vi "Set Workbook.vi"(8 "error in (no error)":errorcluster, 10 "Workbook":refnum<k24>, 11 "Excel Legacy in":refnum<class "Excel Legacy.lvclass">) -> (0 "error out":errorcluster, 3 "Excel Legacy out":refnum<class "Excel Legacy.lvclass">)   [LabVIEW 2013, in "Excel Legacy.lvclass"]
uses:
  Excel Legacy.lvclass
  Excel Legacy.lvclass/Excel Legacy.ctl
  C:/PhaeronGit/LVNPOI/Resources/NPOI 2.1.1 dotnet2/NPOI.dll
  Resources/NPOI 2.1.1 dotnet2/NPOI.dll
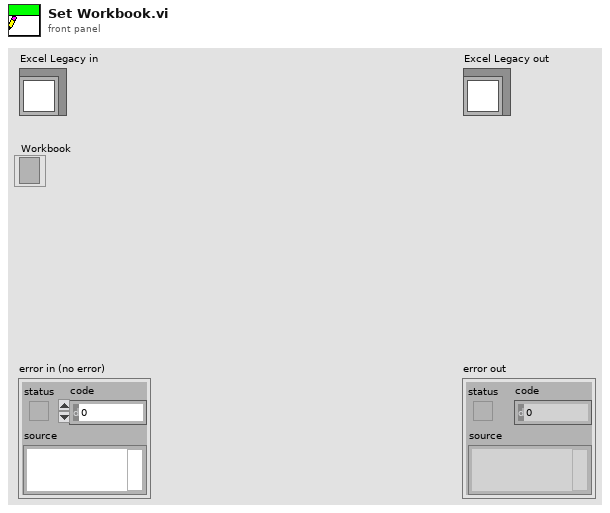
[diagram p1: front panel]
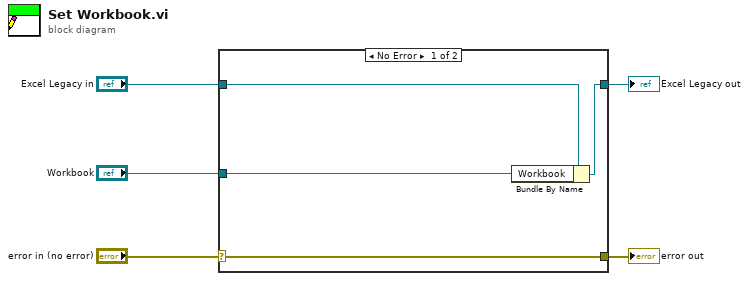
[diagram p0: block diagram]
diagram:
  n1 = case shown="No Error" "error in (no error)" {
    selector: "error in (no error)" -> [w9 w10]
    tunnel: [w9 w10] -> w4
    tunnel: [w7 w11] -> w2
    tunnel: "Excel Legacy in" -> [w8 w11]
    tunnel: "Workbook" -> [w6 _]
    frame No Error {
      n2 = Bundle By Name(cluster=w8, "Workbook"=w6) -> (w7:refnum<class "Excel Legacy.lvclass">)
    }
    frame Error {
    }
  }
  "error out" <- w4
  "Excel Legacy out" <- w2
